vi "DriverStationPushData.vi"   [LabVIEW 2020]
doc: "This VI continously sends data from the robot to the FRC 4265 Dashboard, the joysticks, and the FIRST Driver Station. Data are only sent to the network tables when values change. Detailed sensor data are only sent when the user is currently viewing the Tune tab on the FRC 4265 Dashboard."
uses:
  dsdata.vi
  constants.vi
  <vilib>/Rock Robotics/Network Tables/NT Write String Array.vi
  a59d850d-7f58-4d81-8596-951e7b208772.vi
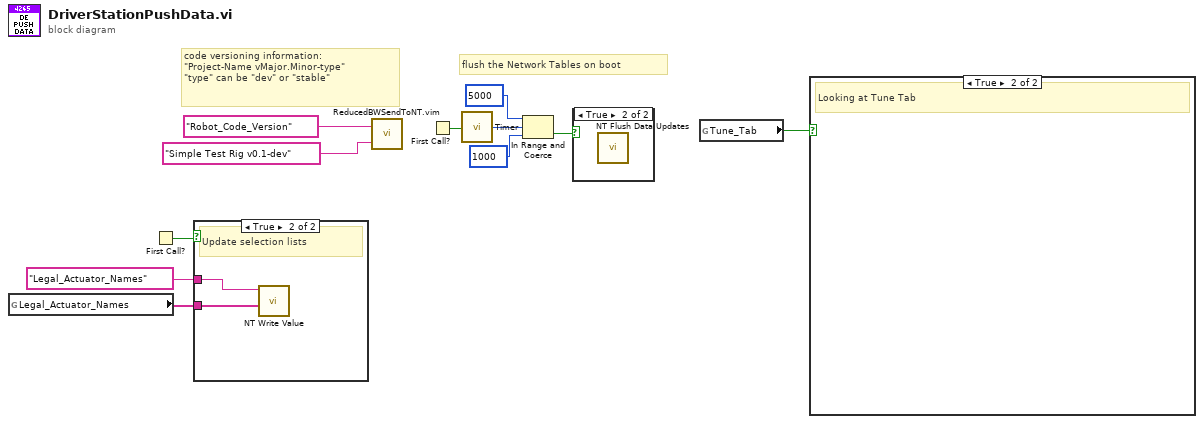
[diagram p0: block diagram]
diagram:
  # "flush the Network Tables on boot"
  # "code versioning information:\n\"Project-Name vMajor.Minor-type\"\n\"type\" can be \"dev\" or \"stable\""
  n1 = global read "constants.vi" "Legal_Actuator_Names"() -> (w10:string[])
  n2 = First Call?() -> (First Call?: T/F=w11:bool)
  n3 = case shown="True" w11 {
    tunnel: w10 -> [_ w13]
    tunnel: "Legal_Actuator_Names" ("Name") -> [_ w12]
    frame False {
    }
    frame True {
      # "Update selection lists"
      n4 = call-poly <vilib>:"NT Write Value.vi"("String Array"=w13, "Name"=w12) -> ()  [unwired: 9 in, 1 out]
    }
  }
  n5 = call "ReducedBWSendToNT.vim"("Value In"="Simple Test Rig v0.1-dev", "NT Name"="Robot_Code_Version" ("Name")) -> ()  [unwired: 1 out]
  n6 = First Call?() -> (First Call?: T/F=w6:bool)
  n7 = call "Timer.vi"("Reset Timer"=w6) -> ("Time (ms)"=w5:u32)
  n8 = In Range and Coerce(upper limit=u32 5000, x=w5, lower limit=u32 1000) -> (In Range?=w2:bool)  [unwired: 1 out]
  n9 = case shown="True" w2 {
    frame False {
    }
    frame True {
      n10 = call <vilib>:"NT Flush Data Updates.vi"() -> ()  [unwired: 11 in, 1 out]
    }
  }
  n11 = global read "dsdata.vi" "Tune_Tab"() -> (w1:bool)
  n12 = case shown="True" w1 {
    frame False {
      # "Not Looking at Tune Tab"
    }
    frame True {
      # "Looking at Tune Tab"
    }
  }
